vi "Prepend Space.vi"(1 "Input String":string) -> (0 "Space + Input String":string)   [LabVIEW 2024]
doc: "This VI inserts a space at the beginning of a string.\nScott Hannahs, FBNML, Jan 1992"
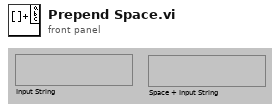
[diagram p1: front panel]
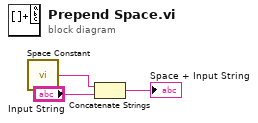
[diagram p0: block diagram]
diagram:
  n1 = call <vilib>:"Space Constant.vi"() -> ("String"=w1:string)
  n2 = Concatenate Strings(w1, "Input String") -> (→"Space + Input String":string)
